vi "1-Integer Detector.vi"() -> ()   [LabVIEW 2014]
panel:
  out "Numeric Indicator 2":dbl
  out "Numeric Indicator":dbl
  out "Integer?":bool
  in  "Number":dbl
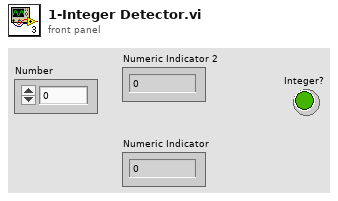
[diagram p1: front panel]
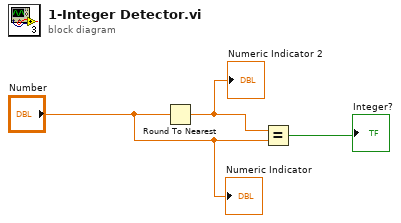
[diagram p0: block diagram]
diagram:
  n1 = Round To Nearest(number="Number") -> (nearest integer value=w2:dbl)
  "Numeric Indicator 2" <- w2
  n2 = Equal?(x=w2, y="Number") -> (x = y?=→"Integer?":bool)
  "Numeric Indicator" <- "Number"
